vi "SetExposure.vi"(8 "error in (no error)":errorcluster, 10 "Setting.Exposure":i32, 11 "Camera_Prime95B in":refnum<class "Camera_Prime95B.lvclass">) -> (0 "error out":errorcluster, 3 "Camera_Prime95B out":refnum<class "Camera_Prime95B.lvclass">)   [LabVIEW 2020, in "Camera_Prime95B.lvlib" / "Camera_Prime95B.lvclass"]
uses:
  Camera_Prime95B.lvclass
  Camera_Prime95B.lvclass/Camera_Prime95B.ctl
  E:/Development/DevHardSoftware/MMicroscopyAF/Model/Real Hardware/Camera_Prime95B/Camera_Prime95B/Dependencies/PVCamNET.dll
  Dependencies/PVCamNET.dll
  HAL Layer/Component/Camera/Camera/Camera.lvclass
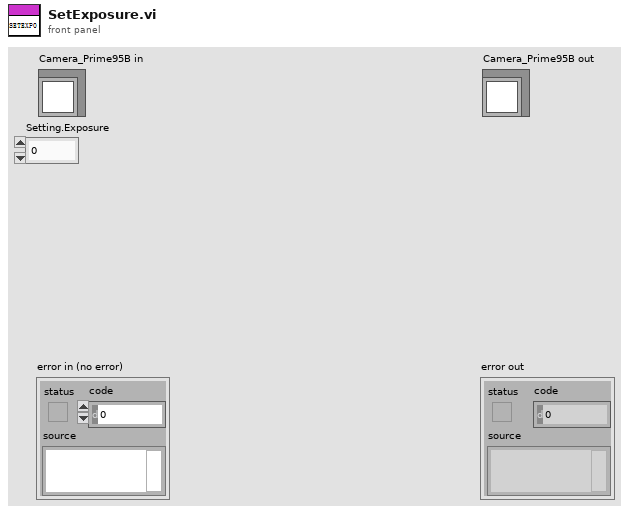
[diagram p1: front panel]
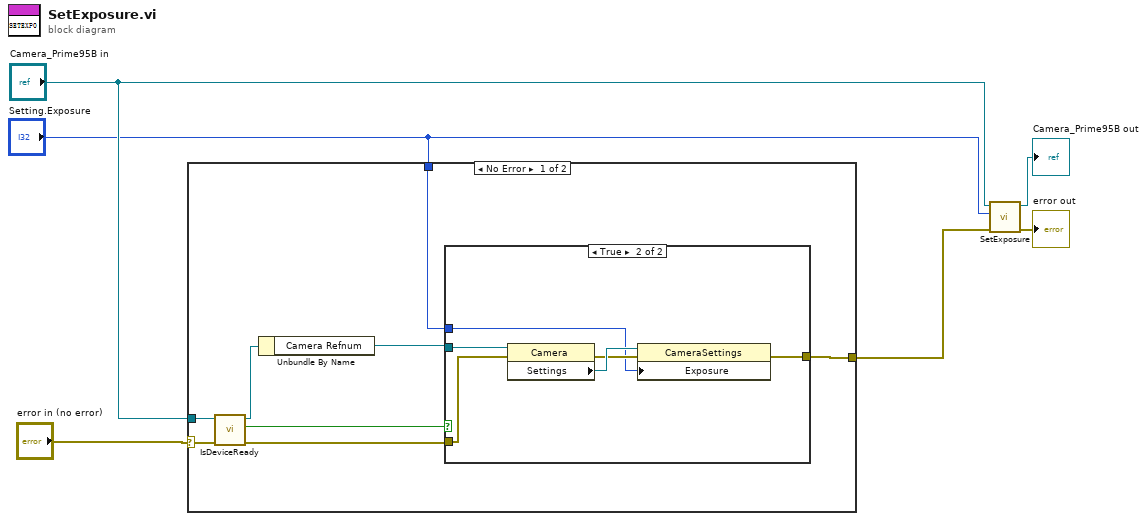
[diagram p0: block diagram]
diagram:
  n1 = case shown="No Error" "error in (no error)" {
    selector: "error in (no error)" -> [w12 w22]
    tunnel: [w13 w22] -> w2
    tunnel: "Camera_Prime95B in" -> [w11 _]
    tunnel: "Setting.Exposure" -> [w14 _]
    frame No Error {
      n2 = call-dynamic "IsDeviceReady.vi"("error in (no error)"=w12, "Camera_Prime95B in"=w11) -> ("error out"=w9:errorcluster, "Ready?"=w10:bool, "Camera_Prime95B out"=w8:refnum<class "Camera_Prime95B.lvclass">)  [unwired: 7 in]
      n3 = Unbundle By Name(w8) -> ("Camera Refnum"=w7:refnum<k24>)
      n4 = case shown="True" w10 {
        tunnel: [w15 w21] -> w13
        tunnel: w7 -> [_ w18]
        tunnel: w14 -> [_ w17]
        tunnel: w9 -> [w15 w16]
        frame False {
        }
        frame True {
          n5 = property class="Camera"(reference=w18, error in=w16) -> (error out=w19:errorcluster, "Settings"=w20:refnum<k24>)  [unwired: 1 out]
          n6 = property class="CameraSettings"(reference=w20, error in=w19, "Exposure"=w17) -> (error out=w21:errorcluster)  [unwired: 1 out]
        }
      }
    }
    frame Error {
    }
  }
  n7 = call-parent "SetExposure.vi"("error in (no error)"=w2, "Setting.Exposure"="Setting.Exposure", "Camera in"="Camera_Prime95B in") -> ("error out"=→"error out":errorcluster, "Camera out"=→"Camera_Prime95B out":refnum<class "Camera_Prime95B.lvclass">)  [unwired: 7 in]
